vi "Config Procces.vi"(0 "reference in":refnum<class "Proccess.lvclass">, 5 "error in (no error)":errorcluster, 6 "Name":string, 8 "ParentName":string, 10 "Description":string, 11 "Logger":refnum<class "Logger.lvclass">) -> (14 "reference out":refnum<class "Proccess.lvclass">, 19 "error out":errorcluster)   [LabVIEW 2019, in "Proccess.lvclass"]
doc: "Constructor."
uses:
  Proccess.lvclass
  Logger_class/ObjType.ctl
  Logger_class/Logger.lvclass
  Logger_class/ObjData.ctl
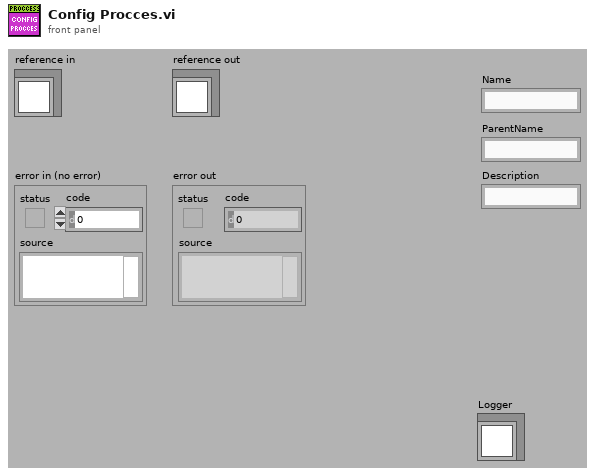
[diagram p1: front panel]
types:
  T1 = typedef "Logger.lvclass/ObjType.ctl" = enum16{"Procces", "Device", "SignalA", "SignalD", "DI", "DO", "DA", "AI", "AO", "AA", "GUI"}
  T2 = typedef "Logger.lvclass/ObjData.ctl" = cluster{"object_tag":string, "parent_tag":string, "object_type":T1, "description":string}
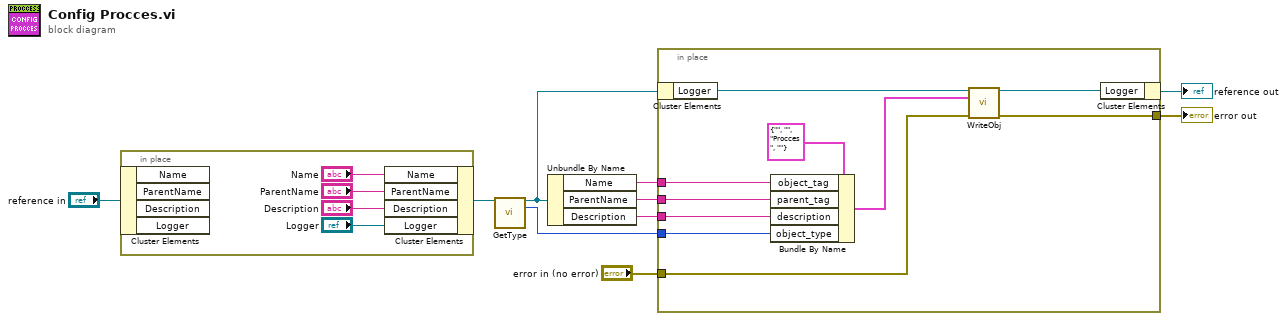
[diagram p0: block diagram]
diagram:
  n1 = in-place {
    n2 = in-place-cluster #1("reference in") -> ()  [unwired: 4 out]
    n3 = in-place-cluster #1("Name"="Name", "ParentName"="ParentName", "Description"="Description", "Logger"="Logger") -> (w8:refnum<class "Proccess.lvclass">)
  }
  n4 = call-dynamic "GetType.vi"("reference in"=w8) -> ("reference out"=w4:refnum<class "Proccess.lvclass">, "obj_type"=w5:T1)  [unwired: 13 in]
  n5 = Unbundle By Name(w4) -> ("Name"=w7:string, "ParentName"=w6:string, "Description"=w3:string)
  n6 = in-place {
    in-place-border: w7 -> [w20]
    in-place-border: w6 -> [w19]
    in-place-border: w5 -> [w18]
    in-place-border: w3 -> [w17]
    in-place-border: "error in (no error)" -> [w16]
    in-place-border: [w15] -> w2
    n7 = in-place-cluster #2(w4) -> ("Logger"=w23:refnum<class "Logger.lvclass">)
    n8 = Bundle By Name(cluster=T2 {"object_tag"="", "parent_tag"="", "object_type"=enum."Procces", "description"=""} ("device"), "object_tag"=w20, "parent_tag"=w19, "description"=w17, "object_type"=w18) -> (w21:T2)
    n9 = call "WriteObj.vi"("reference in"=w23, "device"=w21, "error in (no error)"=w16) -> ("reference out"=w22:refnum<class "Logger.lvclass">, "error out"=w15:errorcluster)  [unwired: 11 in]
    n10 = in-place-cluster #2("Logger"=w22) -> (→"reference out":refnum<class "Proccess.lvclass">)
  }
  "error out" <- w2
